vi "Destroy.vi"(0 "reference in":refnum<class "ACIR_EIS.lvclass">, 5 "Error In":errorcluster) -> (14 "reference out":refnum<class "ACIR_EIS.lvclass">, 19 "Error Out":errorcluster)   [LabVIEW 2023, in "ACIR_EIS.lvclass"]
uses:
  ACIR_EIS.lvclass
  ACIR_EIS.lvclass/ACIR_EIS.ctl
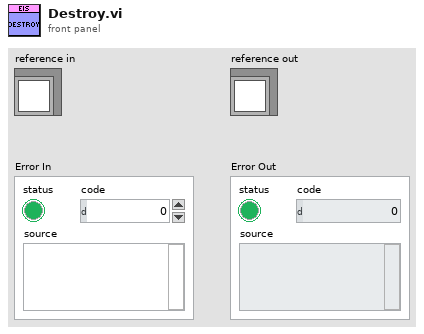
[diagram p1: front panel]
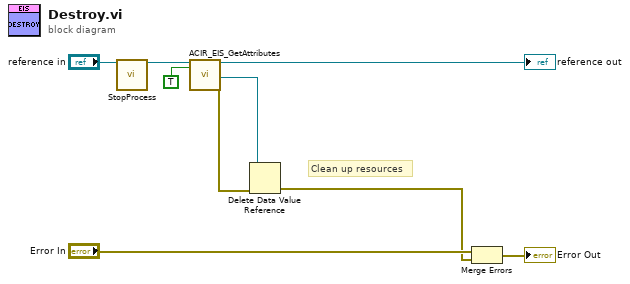
[diagram p0: block diagram]
diagram:
  # "Clean up resources"
  n1 = call "StopProcess.vi"("reference in"="reference in") -> ("reference out"=w1:refnum<class "ACIR_EIS.lvclass">)  [unwired: 17 in, 1 out]
  n2 = call "ACIR_EIS_GetAttributes.vi"("reference in"=w1, "OnlyGetDvrReference(False)"=TRUE) -> ("reference out"=→"reference out":refnum<class "ACIR_EIS.lvclass">, "DataRef"=w6:refnum<data-value>, "Error Out"=w7:errorcluster)  [unwired: 14 in, 1 out]
  n3 = Delete Data Value Reference(data value reference=w6, error in=w7) -> (error out=w4:errorcluster)  [unwired: 1 out]
  n4 = Merge Errors("Error In", w4) -> (→"Error Out":errorcluster)
